vi "Circular Buffer subVI.vi"(6 "History Length [1024]":i32, 7 "Reset":bool, 10 "Buffer in":dbl[](array[numeric]), 11 "Array in":dbl[](array[numeric])) -> (2 "Buffer out":dbl[](array[numeric]), 3 "Array out":dbl[](array[numeric]))   [LabVIEW 2019, in "xy_utilities.lvlib"]
uses:
  xy_utilities.lvlib
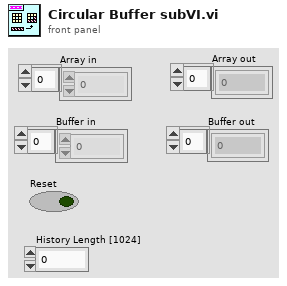
[diagram p1: front panel]
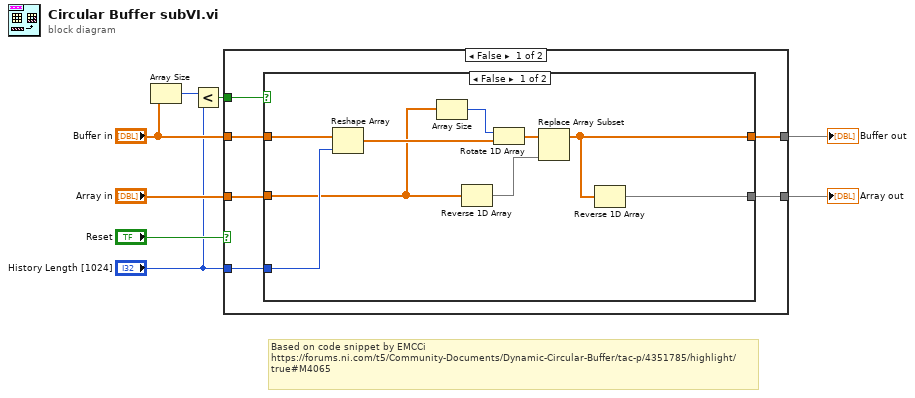
[diagram p0: block diagram]
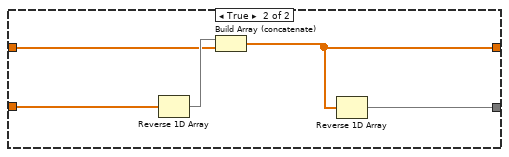
[diagram p2: hidden frame]
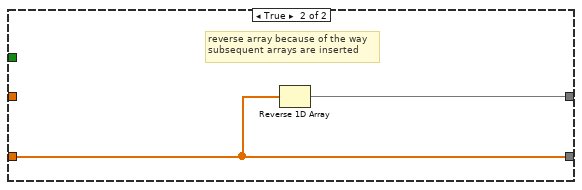
[diagram p3: hidden frame]
diagram:
  # "Based on code snippet by EMCCi\nhttps://forums.ni.com/t5/Community-Documents/Dynamic-Circular-Buffer/tac-p/4351785/highlight/true#M4065"
  n1 = Array Size(array="Buffer in") -> (size(s)=w1:i32)
  n2 = Less?(x=w1, y="History Length [1024]") -> (x < y?=w3:bool)
  n3 = case shown="False" "Reset" {
    tunnel: "Array in" -> [w10 w30]
    tunnel: "History Length [1024]" -> [w14 _]
    tunnel: w3 -> [w13 _]
    tunnel: [w12 w29] -> w7
    tunnel: [w11 w30] -> w6
    tunnel: "Buffer in" -> [w9 _]
    frame False {
      n4 = case shown="False" w13 {
        tunnel: [w20 w24] -> w12
        tunnel: [w18 w28] -> w11
        tunnel: w14 -> [w17 _]
        tunnel: w10 -> [w16 w26]
        tunnel: w9 -> [w15 w25]
        frame False {
          n5 = Reshape Array(w15, w17) -> (w23:dbl[])
          n6 = Array Size(array=w16) -> (size(s)=w19:i32)
          n7 = Reverse 1D Array(array=w16) -> (reversed array=w21:dbl[])
          n8 = Rotate 1D Array(1:w23, 2:w19) -> (0:w22:dbl[])
          n9 = Replace Array Subset(array=w22, new element=w21) -> (w20:dbl[])  [unwired: 1 in]
          n10 = Reverse 1D Array(array=w20) -> (reversed array=w18:dbl[])
        }
        frame True {
          n11 = Reverse 1D Array(array=w26) -> (reversed array=w27:dbl[])
          n12 = Build Array (concatenate)(w27, w25) -> (w24:dbl[])
          n13 = Reverse 1D Array(array=w24) -> (reversed array=w28:dbl[])
        }
      }
    }
    frame True {
      # "reverse array because of the way\nsubsequent arrays are inserted"
      n14 = Reverse 1D Array(array=w30) -> (reversed array=w29:dbl[])
    }
  }
  "Buffer out" <- w7
  "Array out" <- w6
